vi "LEBITplc.PubScaleAndOffsetArray.vi"(0 "i ref in":refnum<vi>, 2 "i attribute in":T1, 5 "error in":errorcluster) -> (14 "i ref out":refnum<vi>, 16 "i attribute out":T1, 17 "ScaleServiceID":i32[](array[numeric]), 18 "OffsetServiceID":i32[](array[numeric]), 19 "error out":errorcluster)   [LabVIEW 2014, in "LEBITplc.lvlib"]
uses:
  LEBITplc.lvlib
  LEBITplc.i attribute.ctl
  CSlibraries/UtilityLib/UtilityLib.valueStatus.ctl
  CSlibraries/UtilityLib/UtilityLib.lvlib
  CS_Core/CSSystem/CoreLib/CoreLib.lvlib
  CSlibraries-extern/DimLVEvent/LVDimInterface/LVDimInterface.lvlib
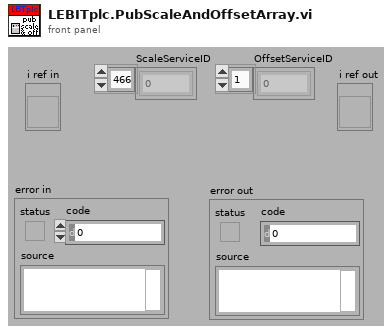
[diagram p1: front panel]
types:
  T1 = typedef "LEBITplc.lvlib/LEBITplc.i attribute.ctl" = cluster{"LLFLocation":string, "SetFileLocation":string, "nickNames":string[], "setValuePLCServiceID":i32[], "GUIServiceID":i32[], "monValuePLC":string[], "SetValueServiceID":i32[], "MonValueServiceID":i32[], "SetValue":dbl[][], "SetValueMin":dbl[], "SetValueMax":dbl[], "SetValueInfoServiceID":i32[], "GUINames":string[], "ListOfBases":string[], "Scale":dbl[], "Offset":dbl[], "setValuePLC":string[], "BaseName":string[], "ScaleServiceID":i32[], "OffsetServiceID":i32[], "AllPLCValues":string[], "CondSpecialArray":string[][], "CondSpecialIndex":i32[], "CondSpecialMonValue":dbl[], "RecentlyChanged":i32[], "SetFileLocationID":i32, "Dependent-Monitors":string[][], "LastLoadedFiles":string[], "IonGuideCalibLocation":string, "Monitor Dependent":string[], "Special":string[], "PLC?":bool[], "Start Date":string, "ListOfBasesServiceID":i32, "SETRA VISA resource":refnum<visa-resource-name>}
  T2 = typedef "UtilityLib.lvlib/UtilityLib.valueStatus.ctl" = enum16{"no info available", "stand by/off", "on", "warning", "alarm/malfunction", "not implemented", "user action required", "important information", "system default", "control default", "indicator default", "button default"}
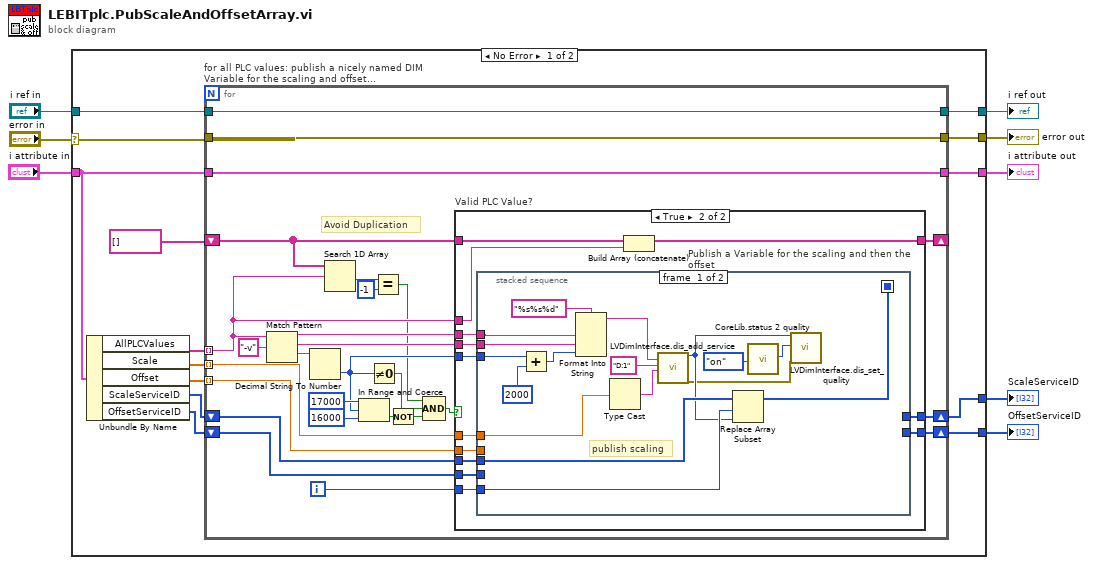
[diagram p0: block diagram]
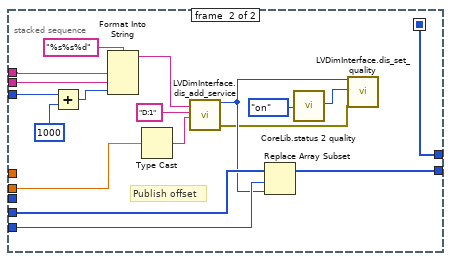
[diagram p3: hidden frame]
diagram:
  n1 = case shown="No Error" "error in" {
    selector: "error in" -> [w19 w102]
    tunnel: "i attribute in" -> [w18 w101]
    tunnel: [w22 w102] -> w7
    tunnel: [w21 w103] -> w6
    tunnel: "i ref in" -> [w20 w103]
    tunnel: [w17 w101] -> w3
    tunnel: [w13 _] -> w2
    tunnel: [w12 _] -> w1
    frame No Error {
      n2 = Unbundle By Name(w18) -> ("AllPLCValues"=w11:string[], "Scale"=w16:dbl[], "Offset"=w15:dbl[], "ScaleServiceID"=w9:i32[], "OffsetServiceID"=w14:i32[])
      n3 = for "for all PLC values: publish a nicely named DIM Variable for the scaling and offset..." {
        tunnel: w20 -> [w49]
        tunnel: w19 -> [w48]
        tunnel: [w48] -> w22
        tunnel: [w49] -> w21
        tunnel: w18 -> [w47]
        tunnel: [w47] -> w17
        tunnel: w11 -> [w31] mode=indexing
        tunnel: w16 -> [w23] mode=indexing
        tunnel: w15 -> [w46] mode=indexing
        shift-right: [w34] -> w13
        shift-left: w9 -> [w45]
        shift-right: [w43] -> w12
        shift-left: w14 -> [w44]
        shift-right: [w33] -> _
        shift-left: string[] [] ("AllPLCValues") -> [w32]
        i -> [w35]
        # "Avoid Duplication"
        n4 = Match Pattern(string=w31, regular expression="-v") -> (before substring=w38:string, match substring=w37:string, after substring=w41:string)  [unwired: 1 in, 1 out]
        n5 = Decimal String To Number(string=w41) -> (number=w36:i32)  [unwired: 2 in, 1 out]
        n6 = Search 1D Array(1D array=w32, element=w31) -> (index of element=w30:i32)  [unwired: 1 in]
        n7 = In Range and Coerce(upper limit=17000 ("lower limit"), x=w36, lower limit=16000 ("upper limit")) -> (In Range?=w25:bool)  [unwired: 1 out]
        n8 = Not Equal To 0?(x=w36) -> (x != 0?=w27:bool)
        n9 = Equal?(x=w30, y=-1) -> (x = y?=w26:bool)
        n10 = Not(x=w25) -> (.not. x?=w24:bool)
        n11 = Compound Arithmetic op=AND(w26, w27, w24) -> (w28:bool)
        n12 = case "Valid PLC Value?" shown="True" w28 {
          tunnel: w46 -> [_ w65]
          tunnel: w45 -> [w52 w64]
          tunnel: w44 -> [w51 w63]
          tunnel: [w52 w62] -> w34
          tunnel: [w51 w61] -> w43
          tunnel: w38 -> [_ w60]
          tunnel: w37 -> [_ w59]
          tunnel: w36 -> [_ w58]
          tunnel: w35 -> [_ w57]
          tunnel: w23 -> [_ w56]
          tunnel: w32 -> [w50 w55]
          tunnel: [w50 w53] -> w33
          tunnel: w31 -> [_ w54]
          frame False {
            # "Invalid or duplicate PLC Value"
          }
          frame True {
            n13 = stacked-sequence "Publish a Variable for the scaling and then the offset" {
              seq-local: [w77 _] -> [_ w94]
              tunnel: w58 -> [w82 w100]
              tunnel: w60 -> [w81 w99]
              tunnel: w59 -> [w80 w98]
              tunnel: w56 -> [w79 _]
              tunnel: w65 -> [_ w97]
              tunnel: w64 -> [w78 _]
              tunnel: [_ w95] -> w61
              tunnel: w63 -> [_ w96]
              tunnel: [_ w94] -> w62
              tunnel: w57 -> [w76 w93]
              frame #0 {
                # "publish scaling"
                n14 = Add(x=w82, y=2000) -> (x+y=w69:i32)
                n15 = Format Into String(format string="%s%s%d", w81, w80, w69) -> (resulting string=w68:string)  [unwired: 2 in, 1 out]
                n16 = Type Cast(x=w79) -> (*(type *) &x=w71:string)  [unwired: 1 in]
                n17 = call "LVDimInterface.dis_add_service.vi"("serviceName"=w68, "typeDescriptor"="D:1", "data"=w71) -> ("my_serviceID"=w73:i32, "error out"=w66:errorcluster)  [unwired: 15 in]
                n18 = Replace Array Subset(array=w78, new element=w73, index=w76) -> (w77:i32[])
                n19 = call "CoreLib.status 2 quality.vi"("valueStatus"=UtilityLib.valueStatus."on") -> ("quality"=w75:i32)  [unwired: 18 in]
                n20 = call "LVDimInterface.dis_set_quality.vi"("my_serviceID"=w73, "quality"=w75, "error in (no error)"=w66) -> ()  [unwired: 15 in, 2 out]
              }
              frame #1 {
                # "Publish offset"
                n21 = Add(x=w100, y=1000) -> (x+y=w86:i32)
                n22 = Format Into String(format string="%s%s%d", w99, w98, w86) -> (resulting string=w85:string)  [unwired: 2 in, 1 out]
                n23 = Type Cast(x=w97) -> (*(type *) &x=w88:string)  [unwired: 1 in]
                n24 = call "LVDimInterface.dis_add_service.vi"("serviceName"=w85, "typeDescriptor"="D:1", "data"=w88) -> ("my_serviceID"=w90:i32, "error out"=w83:errorcluster)  [unwired: 15 in]
                n25 = Replace Array Subset(array=w96, new element=w90, index=w93) -> (w95:i32[])
                n26 = call "CoreLib.status 2 quality.vi"("valueStatus"=UtilityLib.valueStatus."on") -> ("quality"=w92:i32)  [unwired: 18 in]
                n27 = call "LVDimInterface.dis_set_quality.vi"("my_serviceID"=w90, "quality"=w92, "error in (no error)"=w83) -> ()  [unwired: 15 in, 2 out]
              }
            }
            n28 = Build Array (concatenate)(w55, w54) -> (w53:string[])
          }
        }
      }
    }
    frame Error {
    }
  }
  "error out" <- w7
  "i ref out" <- w6
  "i attribute out" <- w3
  "ScaleServiceID" <- w2
  "OffsetServiceID" <- w1
